vi "Database Insert Record.vi"(8 "error in (no error)":errorcluster, 9 "Requesting Module":T4, 10 "Step Data":T3, 11 "Status":T5) -> (0 "error out":errorcluster, 3 "Status":T5)   [LabVIEW 2012]
doc: "Allows the application to insert records into the database"
uses:
  Architecture/Message Queue/Message Cluster.ctl
  Architecture/Message Queue/Message Queue.lvlib
  Car Wash Controller/Controls/Steps.ctl
  Car Wash Controller/Controls/Stations.ctl
  Architecture/Modules.ctl
  Controls/Database Status.ctl
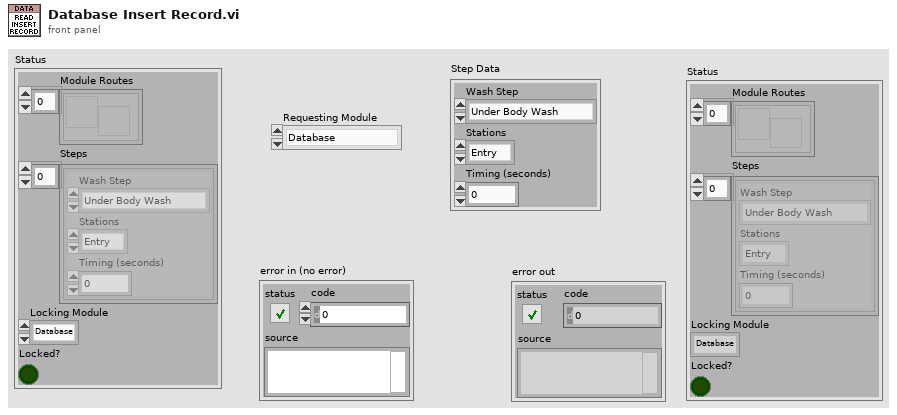
[diagram p1: front panel]
types:
  T1 = typedef "Steps.ctl" = enum16{"Under Body Wash", "Bug Remover", "Pre-Soak", "High Pressure Wash", "Low Pressure Wax", "Spot Free Rinse", "Tire Shine Foam", "Air Dry"}
  T2 = typedef "Stations.ctl" = enum16{"Entry", "Station 1", "Station 2", "Station 3", "Exit"}
  T3 = cluster{"Wash Step":T1, "Stations":T2, "Timing (seconds)":u32}
  T4 = typedef "Modules.ctl" = enum16{"Database", "Car Wash Controller", "Console"}
  T5 = typedef "Database Status.ctl" = cluster{"Module Routes":refnum<user-event>[], "Steps":cluster{"Wash Step":T1, "Stations":T2, "Timing (seconds)":u32}[], "Locking Module":T4, "Locked?":bool}
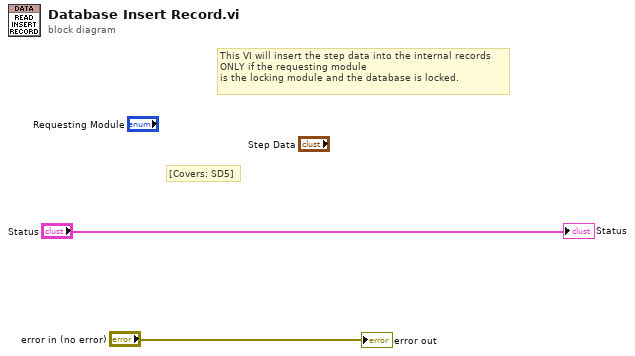
[diagram p0: block diagram]
diagram:
  # "[Covers: SD5]"
  # "This VI will insert the step data into the internal records\nONLY if the requesting module\nis the locking module and the database is locked."
  "error out" <- "error in (no error)"
  "Status" <- "Status"
